vi "SendClusterServerSide.vi"() -> ()   [LabVIEW 2019]
panel:
  in  "Stop from Server Side":bool
  in  "Data Cluster":T1
  out "error out":errorcluster
  out "Side":string
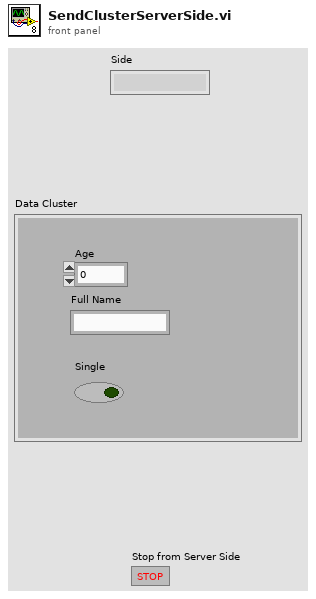
[diagram p1: front panel]
types:
  T1 = cluster{"Age":dbl, "Full Name ":string, "Single":bool}
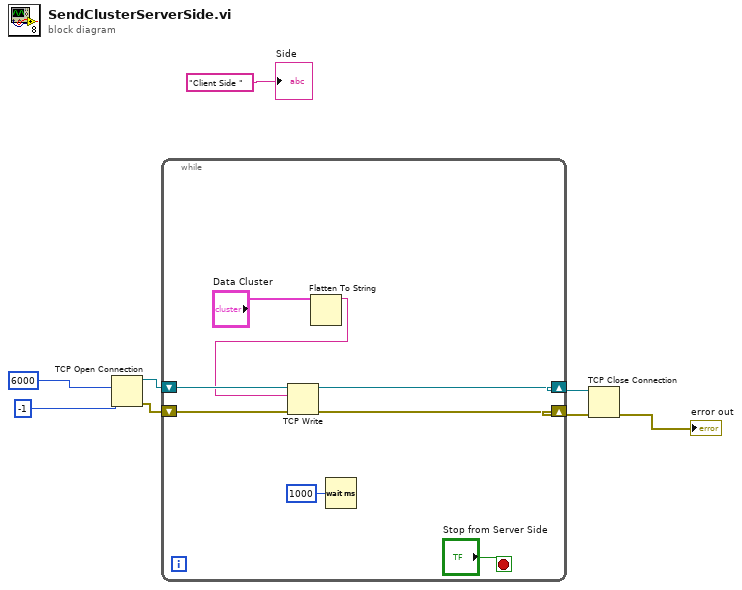
[diagram p0: block diagram]
diagram:
  n1 = TCP Open Connection(remote port or service name=u16 6000, timeout ms (60000)=-1) -> (connection ID=w5:refnum<k5>, error out=w3:errorcluster)  [unwired: 3 in]
  n2 = while {
    shift-right: [w15] -> w4
    shift-left: w5 -> [w16]
    shift-right: [w13] -> w2
    shift-left: w3 -> [w14]
    stop <- "Stop from Server Side" stop-if-true
    n3 = Flatten To String(anything="Data Cluster") -> (data string=w11:string)  [unwired: 3 in, 2 out]
    n4 = TCP Write(connection ID=w16, data in=w11, error in (no error)=w14) -> (connection ID out=w15:refnum<k5>, error out=w13:errorcluster)  [unwired: 1 in, 1 out]
    n5 = Wait (ms)(milliseconds to wait=u32 1000) -> ()  [unwired: 1 out]
  }
  n6 = TCP Close Connection(connection ID=w4, error in (no error)=w2) -> (error out=→"error out":errorcluster)  [unwired: 1 in, 1 out]
  "Side" <- "Client Side " ("String")
